vi "Tarea2.vi"() -> ()   [LabVIEW 2025]
uses:
  <vilib>/express/express analysis/Spectral/Block/exnSpectralBlock spectral measurements power poly.vi
  <vilib>/express/express analysis/Spectral/Block/exnSpectralBlock spectral measurements power DDT.vi
  <vilib>/express/express analysis/Spectral/XNode/ExpressSpectralMeasurementsBlockNode.xnode
panel:
  out "Waveform Graph 3":dynamicdata(graph)
  out "Sine 2":dynamicdata(graph) caption="Sine"
  out "Sine":dynamicdata(graph)
  out "Waveform Graph 2":dynamicdata(graph)
  out "Waveform Graph":dynamicdata(graph)
  in  "stop":bool
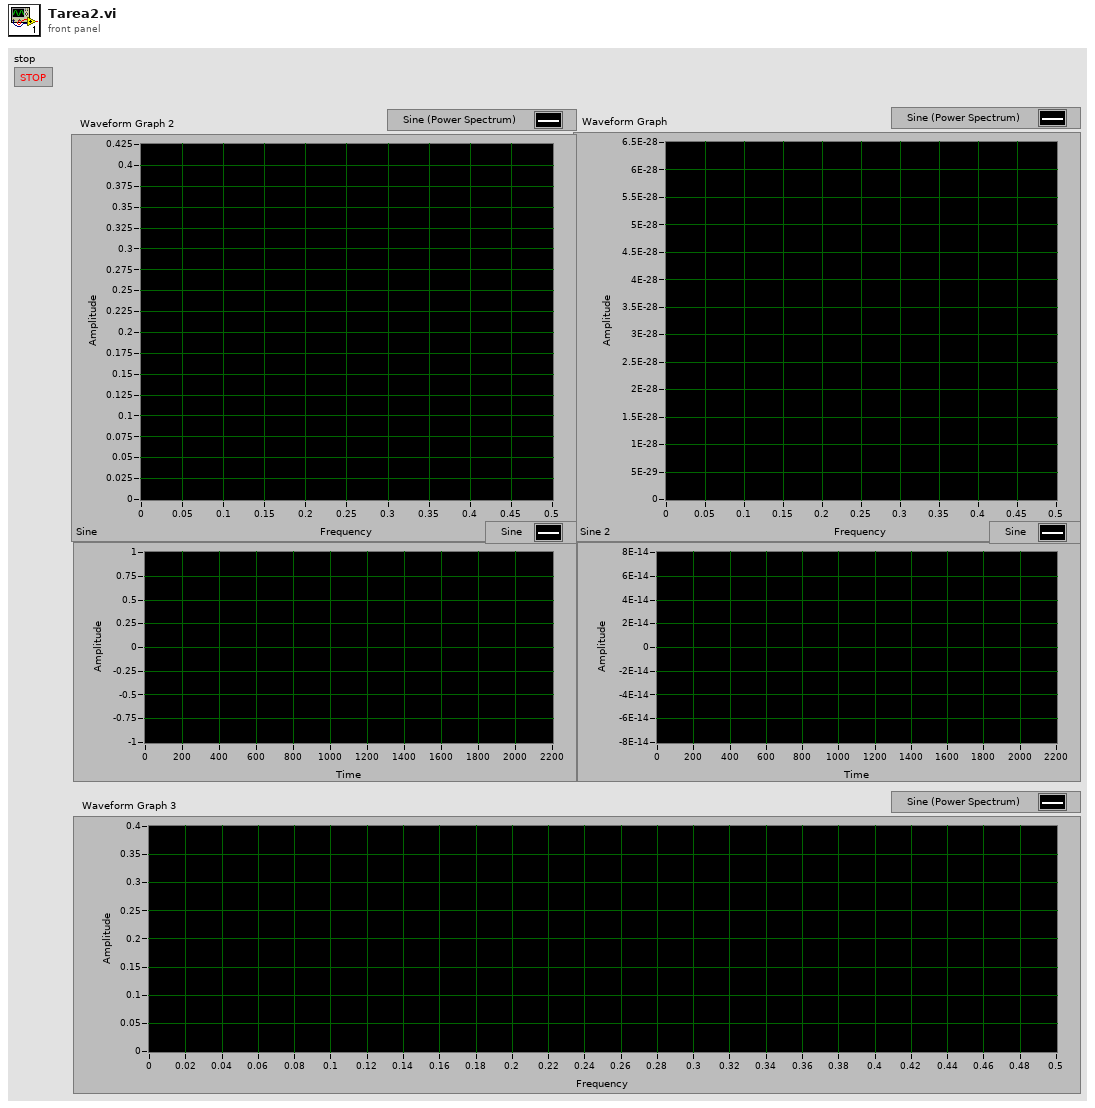
[diagram p1: front panel]
types:
  T1 = cluster{"averaging mode":u16, "weighting mode":u16, "number of averages":u32}
  T2 = cluster{"dB On (F)":bool, "unwrap phase (F)":bool, "convert to degree (F)":bool}
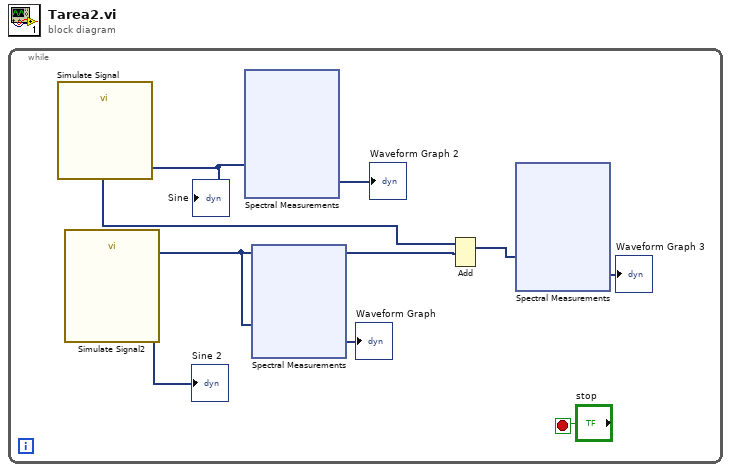
[diagram p0: block diagram]
diagram:
  n1 = while {
    stop <- "stop" stop-if-true
    n2 = call "Simulate Signal"() -> ("Sine"=w4:dynamicdata)  [unwired: 14 in, 1 out]
    "Sine" <- w4
    n3 = call "Simulate Signal2"() -> ("Sine"=w3:dynamicdata)  [unwired: 14 in, 1 out]
    "Sine 2" <- w3
    n4 = xnode "Spectral Measurements"("Signals"=w4) -> ("Power Spectrum"=→"Waveform Graph 2":dynamicdata)  [unwired: 1 in, 1 out]
    n5 = xnode "Spectral Measurements"("Signals"=w3) -> ("Power Spectrum"=→"Waveform Graph":dynamicdata)  [unwired: 1 in, 1 out]
    n6 = Add(1:w3, 2:w4) -> (0:w2:dynamicdata)  [unwired: 1 in, 1 out]
    n7 = xnode "Spectral Measurements"("Signals"=w2) -> ("Power Spectrum"=→"Waveform Graph 3":dynamicdata)  [unwired: 1 in, 1 out]
  }
